vi "Get Force Table Entry.vi"(8 "error in (no error)":errorcluster, 11 "Model in":refnum<class "Model.lvclass">) -> (0 "error out":errorcluster, 2 "Entry":T1[](array[typedef]) {"Axial Force" format="%.4f"; "Lateral Force" format="%.4f"}, 3 "Model out":refnum<class "Model.lvclass">)   [LabVIEW 2016]
uses:
  Typedefs/ForcePair.ctl
  Model.lvclass
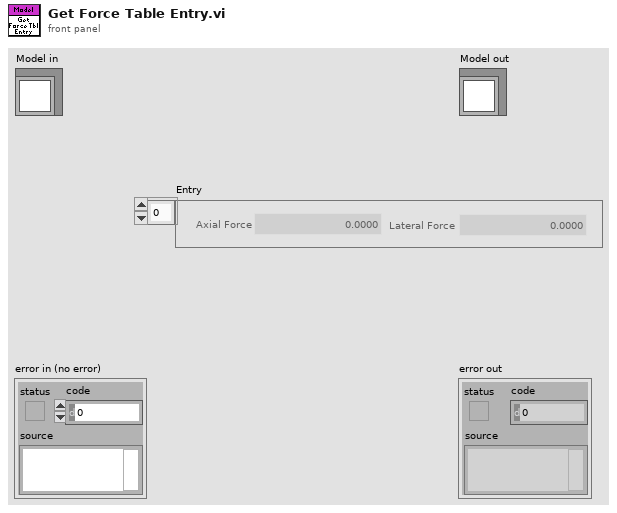
[diagram p1: front panel]
types:
  T1 = typedef "ForcePair.ctl" = cluster{"Axial Force":dbl, "Lateral Force":dbl}
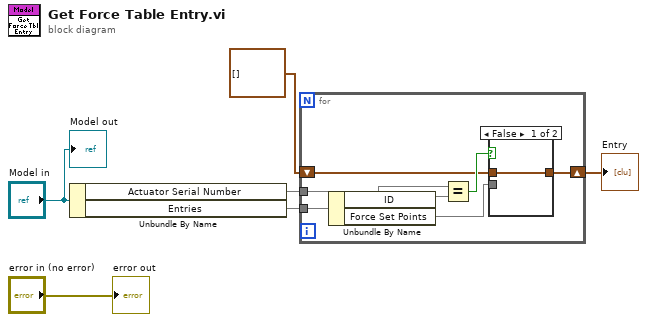
[diagram p0: block diagram]
diagram:
  n1 = Unbundle By Name("Model in") -> ("Actuator Serial Number"=w5, "Entries"=w6)
  n2 = for {
    tunnel: w6 -> [w13]
    tunnel: w5 -> [w12]
    shift-right: [w8] -> w3
    shift-left: T1[] [] -> [w7]
    n3 = Unbundle By Name(w13) -> ("ID"=w11, "Force Set Points"=w9)
    n4 = Equal?(x=w12, y=w11) -> (x = y?=w10:bool)
    n5 = case shown="False" w10 {
      tunnel: w9 -> [_ w15]
      tunnel: [w14 w15] -> w8
      tunnel: w7 -> [w14 _]
      frame False {
      }
      frame True {
      }
    }
  }
  "Entry" <- w3
  "error out" <- "error in (no error)"
  "Model out" <- "Model in"
